vi "PRIME Detector Read Exposure Frames.vi"(11 "Exp Frames":T2) -> (3 "Images":T1[](array[typedef]) {"Detector #" items=["None", "YJ", "HK"]})   [LabVIEW 2024, in "PRIME Detector.lvclass"]
uses:
  PRIME Detector.lvclass
  Detector Image typedef cluster.ctl
  Detector Class.lvclass
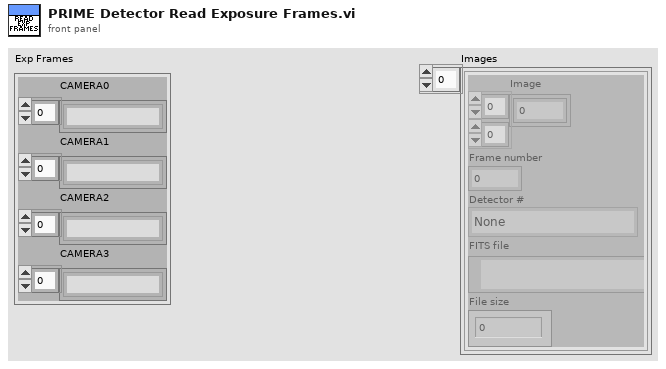
[diagram p1: front panel]
types:
  T1 = typedef "Detector Class.lvclass/Detector Image typedef cluster.ctl" = cluster{"Image":sgl[][], "Frame number":i32, "Detector #":u16, "FITS file":path, "File size":i64}
  T2 = cluster{"CAMERA0":string[], "CAMERA1":string[], "CAMERA2":string[], "CAMERA3":string[]}
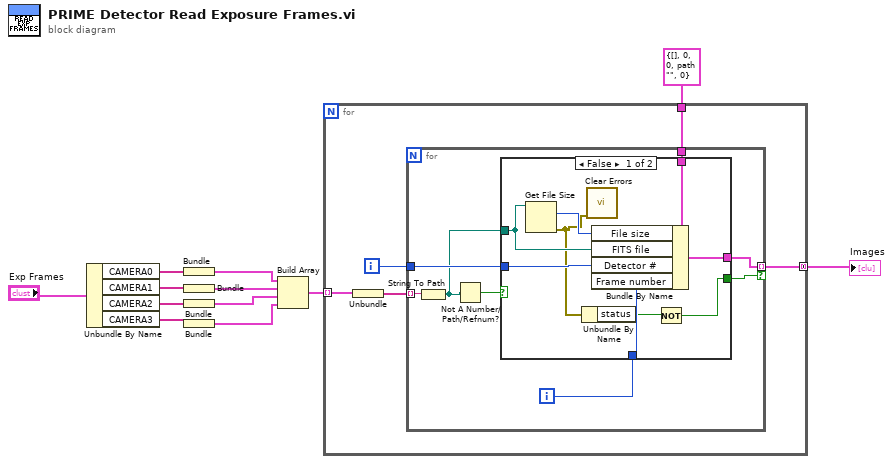
[diagram p0: block diagram]
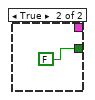
[diagram p2: hidden frame]
diagram:
  n1 = Unbundle By Name("Exp Frames") -> ("CAMERA0"=w11:string[], "CAMERA1"=w8:string[], "CAMERA2"=w10:string[], "CAMERA3"=w9:string[])
  n2 = Bundle("CAMERA0"=w11) -> (w7:cluster{"CAMERA0":string[]})  [unwired: 1 in]
  n3 = Bundle("CAMERA1"=w8) -> (w6:cluster{"CAMERA1":string[]})  [unwired: 1 in]
  n4 = Bundle("CAMERA2"=w10) -> (w5:cluster{"CAMERA2":string[]})  [unwired: 1 in]
  n5 = Bundle("CAMERA3"=w9) -> (w4:cluster{"CAMERA3":string[]})  [unwired: 1 in]
  n6 = Build Array(w7, w6, w5, w4) -> (w3:cluster{"CAMERA3":string[]}[])
  n7 = for {
    tunnel: T1 {"Image"=[], "Frame number"=0, "Detector #"=0, "FITS file"=path "", "File size"=0} ("Image Data") -> [w14]
    tunnel: w3 -> [w17] mode=indexing
    tunnel: [w13] -> w2 mode=concatenating
    i -> [w15]
    n8 = Unbundle(w17) -> ("CAMERA3"=w16:string[])
    n9 = for {
      tunnel: w16 -> [w25] mode=indexing
      tunnel: w14 -> [w24]
      tunnel: w15 -> [w22]
      tunnel: [w21] -> w13 mode=indexing if=w18
      i -> [w23]
      n10 = String To Path(string=w25) -> (path=w20:path)
      n11 = Not A Number/Path/Refnum?(number/path/refnum=w20) -> (NaN/Path/Refnum?=w19:bool)
      n12 = case shown="False" w19 {
        tunnel: w24 -> [w34 _]
        tunnel: w23 -> [w33 _]
        tunnel: w22 -> [w32 _]
        tunnel: [w30 _] -> w21
        tunnel: w20 -> [w29 _]
        tunnel: [w26 FALSE] -> w18
        frame False {
          n13 = Get File Size(file=w29) -> (size (in bytes)=w31:i64, 0:w28:errorcluster)  [unwired: 1 in, 1 out]
          n14 = Unbundle By Name(w28) -> ("status"=w27:bool)
          n15 = call <vilib>:"Clear Errors.vi"("error in (no error)"=w28) -> ()  [unwired: 5 in, 2 out]
          n16 = Bundle By Name(cluster=w34, "File size"=w31, "FITS file"=w29, "Detector #"=w32, "Frame number"=w33) -> (w30:T1)
          n17 = Not(x=w27) -> (.not. x?=w26:bool)
        }
        frame True {
        }
      }
    }
  }
  "Images" <- w2
